vi "Set Cell Color.vi"(8 "error in":errorcluster, 10 "color":u32(colorbox)=16777215, 11 "XLS in":refnum<class "XLS.lvclass">=refnum) -> (0 "error out":errorcluster, 3 "XLS out":refnum<class "XLS.lvclass">)   [LabVIEW 2017, in "Report_lib.lvlib" / "XLS.lvclass"]
doc: "This method set background color\nof cell based on row/column coordinates"
uses:
  XLS.lvclass
  <vilib>/Utility/NIReport.llb/Excel/NI_Excel.lvclass
  <vilib>/Utility/NIReport.llb/NI_report.lvclass
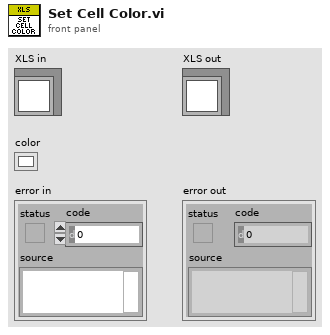
[diagram p1: front panel]
types:
  T1 = cluster{"on/off":bool, "weight":i32, "color":u32}
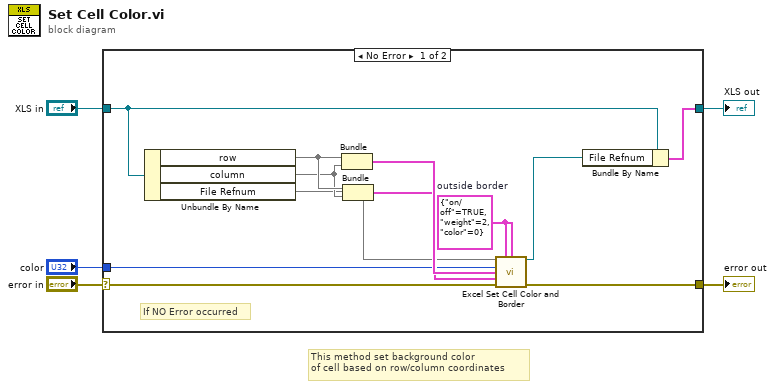
[diagram p0: block diagram]
diagram:
  # "This method set background color\nof cell based on row/column coordinates"
  n1 = case shown="No Error" "error in" {
    selector: "error in" -> [w11 w19]
    tunnel: [w10 w19] -> w4
    tunnel: [w8 w18] -> w2
    tunnel: "XLS in" -> [w9 w18]
    tunnel: "color" -> [w6 _]
    frame No Error {
      w17 = T1 {"on/off"=TRUE, "weight"=2, "color"=0}  # outside border
      # "If NO Error occurred"
      n2 = Unbundle By Name(w9) -> ("row"=w14, "column"=w13, "File Refnum"=w12)
      n3 = Bundle("row"=w14, "column"=w13) -> (w16:cluster{"row":void, "column":void})  [unwired: 1 in]
      n4 = Bundle("row"=w14, "column"=w13) -> (w15:cluster{"row":void, "column":void})  [unwired: 1 in]
      n5 = call <vilib>:"Excel Set Cell Color and Border.vi"("report in"=w12, "inside border"=w17, "outside border"=w17, "background color (w)"=w6, "start (-1, -1)"=w16, "end (-1, -1)"=w15, "error in (no error)"=w11) -> ("report out"=w7:refnum<class "NI_report.lvclass">, "error out"=w10:errorcluster)  [unwired: 7 in]
      n6 = Bundle By Name(cluster=w9, "File Refnum"=w7) -> (w8:cluster{})
    }
    frame Error {
    }
  }
  "error out" <- w4
  "XLS out" <- w2
